vi "PXIe-4139 Initialization - Add DCPower Channel.vi"(8 "error in (no error)":errorcluster, 9 "Channel #":i32, 10 "Channel Name":string, 11 "Device Item Ref In":T1 format="%.0x") -> (0 "error out":errorcluster, 3 "Device Item Ref Out":T1 format="%.0x")   [LabVIEW 2023, in "PXIe-4139 Custom Device.lvlib"]
uses:
  PXIe-4139 Custom Device.lvlib
  <vilib>/NI VeriStand/Custom Device API/Custom Device Item Ref.ctl
  <vilib>/NI VeriStand/Custom Device API/Custom Device Channel Type.ctl
  <vilib>/NI VeriStand/Custom Device API/Custom Device Channel.ctl
  Controls/Channel Type.ctl
  Controls/Channel Sense.ctl
  PXIe-4139 Global Variable.vi
  <vilib>/NI VeriStand/Custom Device API/Set Item Property (I32).vi
  <vilib>/NI VeriStand/Custom Device API/Custom Device API.lvlib
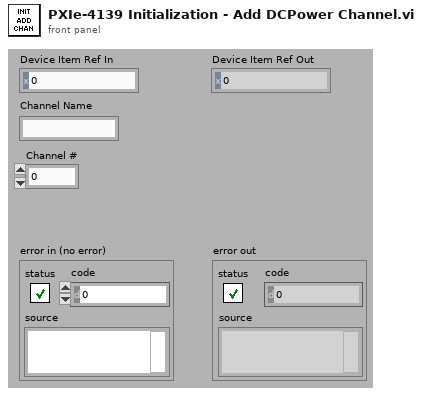
[diagram p1: front panel]
types:
  T1 = typedef "Custom Device API.lvlib/Custom Device Item Ref.ctl" = u64
  T2 = typedef "PXIe-4139 Custom Device.lvlib/Channel Sense.ctl" = i32
  T3 = typedef "PXIe-4139 Custom Device.lvlib/Channel Type.ctl" = i32
  T4 = typedef "Custom Device API.lvlib/Custom Device Channel Type.ctl" = enum16{"Input", "Output"}
  T5 = typedef "Custom Device API.lvlib/Custom Device Channel.ctl" = cluster{"Type":T4, "Units":string, "Default Value":dbl, "Faultable":bool, "Scalable":bool}
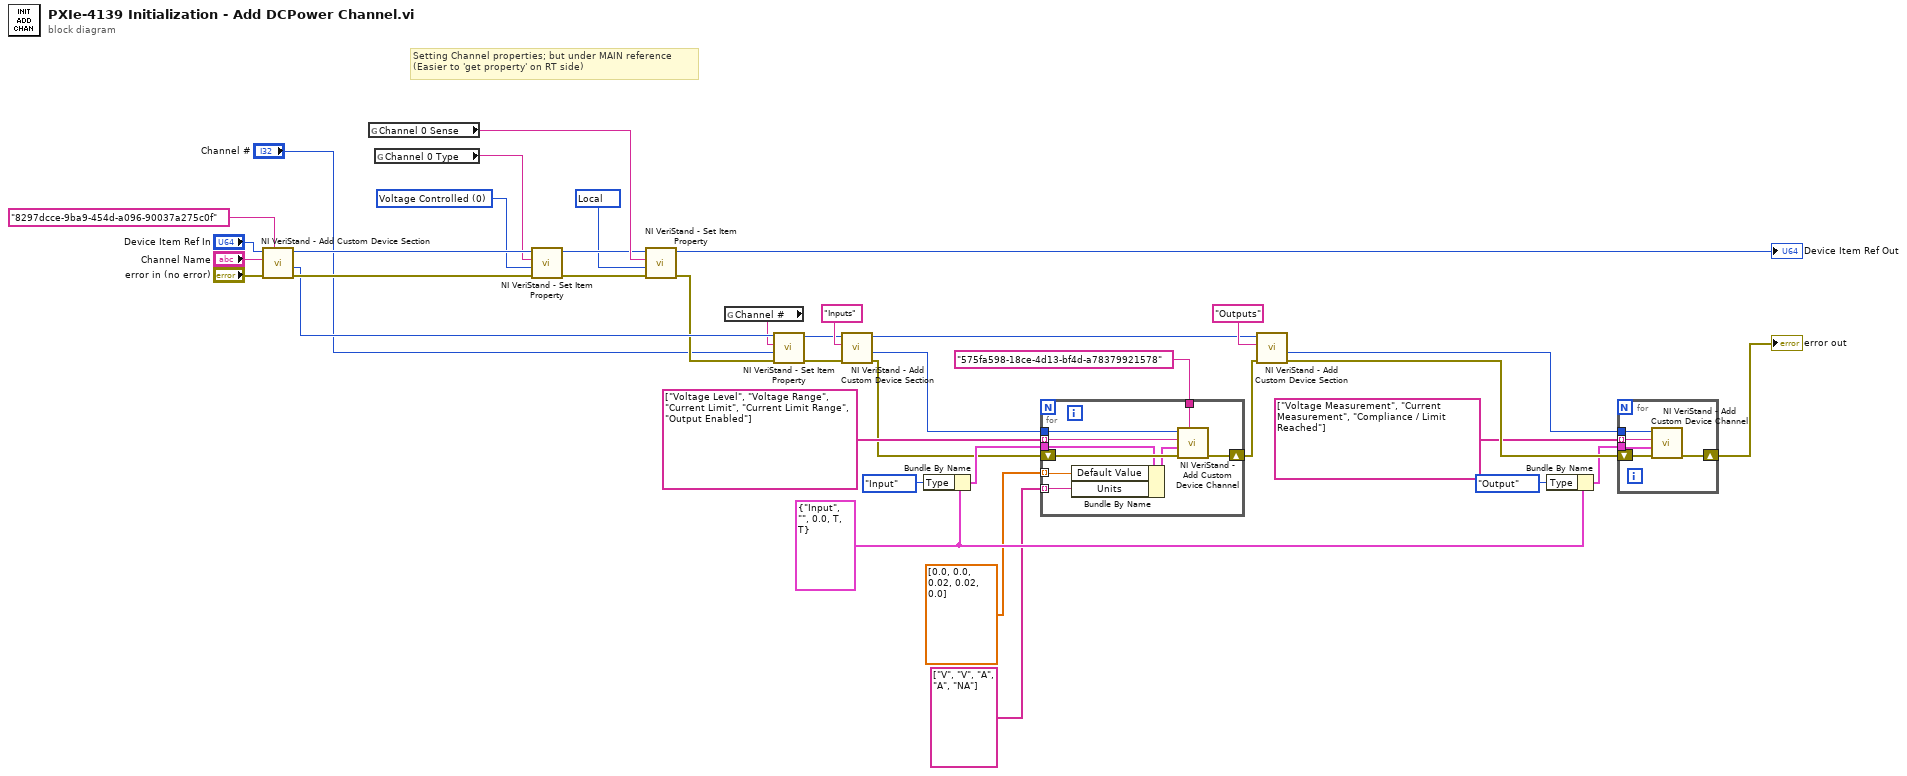
[diagram p0: block diagram]
diagram:
  w4 = T2 1008 items=["Local"=1008, "Remote"=1009] ("Channel Sense")
  w15 = T3 0 items=["Voltage Controlled", "Current Controlled"] ("Channel Type")
  w22 = T5 {"Type"=enum."Input", "Units"="", "Default Value"=0.0, "Faultable"=TRUE, "Scalable"=TRUE} ("Channel")
  # "Setting Channel properties; but under MAIN reference\n(Easier to 'get property' on RT side)"
  n1 = call <vilib>:"NI VeriStand - Add Custom Device Section.vi"("GUID (Default Section)"="8297dcce-9ba9-454d-a096-90037a275c0f", "error in (no error)"="error in (no error)", "Section Name"="Channel Name", "Parent Ref in"="Device Item Ref In") -> ("error out"=w16:errorcluster, "Section Ptr"=w9:T1, "Parent Ref out"=w20:T1)  [unwired: 4 in, 1 out]
  n2 = global read "PXIe-4139 Global Variable.vi" "Channel 0 Sense"() -> (w14:string)
  n3 = global read "PXIe-4139 Global Variable.vi" "Channel 0 Type"() -> (w19:string)
  n4 = call-poly <vilib>:"NI VeriStand - Set Item Property.vi"("error in (no error)"=w16, "Value"=w15, "Property Name"=w19, "Item Ref in"=w20) -> ("error out"=w8:errorcluster, "Item Ref out"=w13:T1)  [unwired: 5 in, 1 out]
  n5 = call-poly <vilib>:"NI VeriStand - Set Item Property.vi"("Value"=w4, "Property Name"=w14, "Item Ref in"=w13) -> ("Item Ref out"=→"Device Item Ref Out":T1)  [unwired: 6 in, 2 out]
  n6 = global read "PXIe-4139 Global Variable.vi" "Channel #"() -> (w6:string)
  n7 = call-poly <vilib>:"NI VeriStand - Set Item Property.vi"("error in (no error)"=w8, "Value"="Channel #", "Property Name"=w6, "Item Ref in"=w9) -> ("error out"=w7:errorcluster, "Item Ref out"=w10:T1)  [unwired: 5 in, 1 out]
  n8 = call <vilib>:"NI VeriStand - Add Custom Device Section.vi"("error in (no error)"=w7, "Section Name"="Inputs", "Parent Ref in"=w10) -> ("error out"=w33:errorcluster, "Section Ptr"=w34:T1, "Parent Ref out"=w18:T1)  [unwired: 5 in, 1 out]
  n9 = Bundle By Name(cluster=w22, "Type"=Custom_Device_Channel_Type."Input") -> (w35:T5)
  n10 = for {
    tunnel: w34 -> [w46]
    tunnel: string[] ["Voltage Level", "Voltage Range", "Current Limit", "Current Limit Range", "Output Enabled"] -> [w44] mode=indexing
    tunnel: w35 -> [w42]
    shift-right: [w43] -> w23
    shift-left: w33 -> [w45]
    tunnel: dbl[] [0.0, 0.0, 0.02, 0.02, 0.0] -> [w40] mode=indexing
    tunnel: string[] ["V", "V", "A", "A", "NA"] -> [w39] mode=indexing
    tunnel: "575fa598-18ce-4d13-bf4d-a78379921578" ("Section Name") -> [w38]
    n11 = Bundle By Name(cluster=w42, "Default Value"=w40, "Units"=w39) -> (w41:T5)
    n12 = call <vilib>:"NI VeriStand - Add Custom Device Channel.vi"("GUID (Default Channel)"=w38, "error in (no error)"=w45, "Channel"=w41, "Channel Name"=w44, "Parent Ref in"=w46) -> ("error out"=w43:errorcluster)  [unwired: 3 in, 3 out]
  }
  n13 = call <vilib>:"NI VeriStand - Add Custom Device Section.vi"("error in (no error)"=w23, "Section Name"="Outputs", "Parent Ref in"=w18) -> ("error out"=w31:errorcluster, "Section Ptr"=w30:T1)  [unwired: 5 in, 2 out]
  n14 = Bundle By Name(cluster=w22, "Type"=Custom_Device_Channel_Type."Output") -> (w29:T5)
  n15 = for {
    tunnel: w30 -> [w51]
    tunnel: string[] ["Voltage Measurement", "Current Measurement", "Compliance / Limit Reached"] -> [w49] mode=indexing
    tunnel: w29 -> [w48]
    shift-right: [w47] -> w21
    shift-left: w31 -> [w50]
    n16 = call <vilib>:"NI VeriStand - Add Custom Device Channel.vi"("error in (no error)"=w50, "Channel"=w48, "Channel Name"=w49, "Parent Ref in"=w51) -> ("error out"=w47:errorcluster)  [unwired: 4 in, 3 out]
  }
  "error out" <- w21
